vi "image string to array for Python.vi"   [LabVIEW 2020]
types:
  T1 = typedef "Image Type" = u32
  T2 = typedef "IMAQ Image.ctl" = refnum<image>
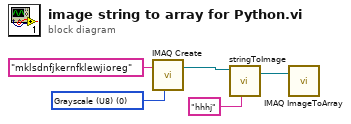
[diagram p0: block diagram]
diagram:
  w4 = T1 0 items=["Grayscale (U8)", "Grayscale (I16)", "Grayscale (SGL)", "Complex (CSG)", "RGB (U32)", "HSL (U32)", "RGB (U64)", "Grayscale (U16)"] ("Image Type")
  n1 = call "IMAQ Create"("Image Name"="mklsdnfjkernfklewjioreg", "Image Type"=w4) -> ("New Image"=w5:T2)  [unwired: 3 in, 1 out]
  n2 = call "stringToImage.vi"("label text (image name)"="hhhj", "Refnum in"=w5) -> ("Refnum out"=w1:T2)  [unwired: 6 in, 3 out]
  n3 = call "IMAQ ImageToArray"("Image"=w1) -> ()  [unwired: 3 in, 5 out]
